vi "PatternCheck.vi"(10 "FullString":string="1312", 11 "Pattern 2":string="12") -> (3 "PatternInString":bool)   [LabVIEW 2025, in "2025_2.lvclass"]
uses:
  2025_2.lvclass
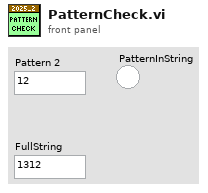
[diagram p1: front panel]
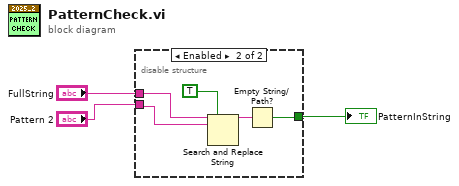
[diagram p0: block diagram]
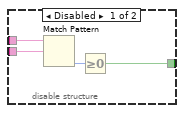
[diagram p2: hidden frame]
diagram:
  n1 = disable-structure shown="Enabled" {
    disable-tunnel: "FullString" -> [w7 w9]
    disable-tunnel: "Pattern 2" -> [w6 w8]
    disable-tunnel: [w4 w10] -> w1
    frame Disabled {
      n2 = Match Pattern(string=w7, regular expression=w6) -> (offset past match=w5:i32)  [unwired: 1 in, 3 out]
      n3 = Greater Or Equal To 0?(x=w5) -> (x >= 0?=w4:bool)
    }
    frame Enabled {
      n4 = Search and Replace String(replace all?=TRUE ("replace all? (F)"), input string=w9, search string=w8) -> (result string=w11:string)  [unwired: 5 in, 3 out]
      n5 = Empty String/Path?(string/path=w11) -> (empty?=w10:bool)
    }
  }
  "PatternInString" <- w1
